vi "ControlReadPulse.vi"(3 "控制电机":T1) -> (1 "PulsOut":i32)   [LabVIEW 2018]
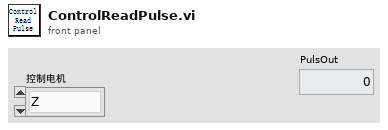
[diagram p1: front panel]
types:
  T1 = typedef "控制电机枚举器.ctl" = enum16{"Z", "Y", "X", "发散角", "俯仰", "旋转"}
  T2 = cluster{"激光器型号":string, "X":dbl, "Y":dbl, "Z":dbl, "Rotate":dbl, "Pitching":dbl, "DivergeAngle":dbl}
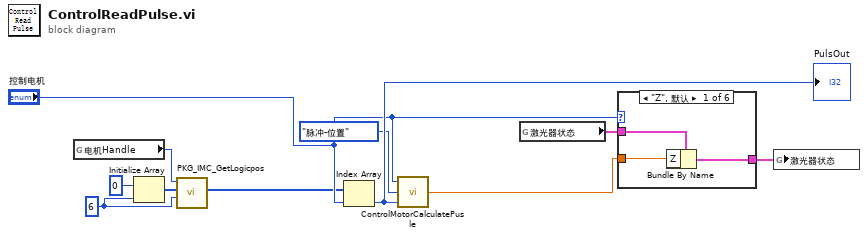
[diagram p0: block diagram]
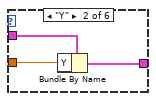
[diagram p2: hidden frame]
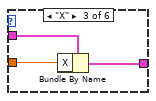
[diagram p3: hidden frame]
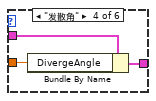
[diagram p4: hidden frame]
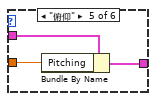
[diagram p5: hidden frame]
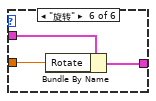
[diagram p6: hidden frame]
diagram:
  w2 = 6 ("维数大小")
  n1 = global read "参数.vi" "电机Handle"() -> (w3:u32)
  n2 = Initialize Array(u32 0 ("元素"), w2) -> (w4:u32[])
  n3 = call "PKG_IMC_GetLogicpos.vi"("axisnum"=w2, "pos"=w4, "Handle"=w3) -> ("pos out"=w1:i32[])  [unwired: 6 in, 2 out]
  n4 = Index Array(array=w1, index="控制电机") -> (element=w10:i32)
  "PulsOut" <- w10
  n5 = call "ControlMotorCalculatePusle.vi"("数据"=w10, "计算状态"=enum32{"位置-脉冲", "脉冲-位置"}."脉冲-位置", "控制电机"="控制电机") -> ("dataout"=w7:dbl)  [unwired: 2 in]
  n6 = global read "参数.vi" "激光器状态"() -> (w8:T2)
  n7 = case shown="\"Z\", 默认" "控制电机" {
    tunnel: w8 -> [w13 w17 w20 w22 w25 w28]
    tunnel: w7 -> [w14 w16 w19 w23 w26 w29]
    tunnel: [w12 w15 w18 w21 w24 w27] -> w6
    frame "Z", Default {
      n8 = Bundle By Name(cluster=w13, "Z"=w14) -> (w12:T2)
    }
    frame "Y" {
      n9 = Bundle By Name(cluster=w17, "Y"=w16) -> (w15:T2)
    }
    frame "X" {
      n10 = Bundle By Name(cluster=w20, "X"=w19) -> (w18:T2)
    }
    frame "发散角" {
      n11 = Bundle By Name(cluster=w22, "DivergeAngle"=w23) -> (w21:T2)
    }
    frame "俯仰" {
      n12 = Bundle By Name(cluster=w25, "Pitching"=w26) -> (w24:T2)
    }
    frame "旋转" {
      n13 = Bundle By Name(cluster=w28, "Rotate"=w29) -> (w27:T2)
    }
  }
  n14 = global write "参数.vi" "激光器状态"(w6) -> ()
